vi "Global 1.vi"() -> ()   [LabVIEW 2018]
panel:
  in  "Alarm Message":string
  out "QUIT":bool
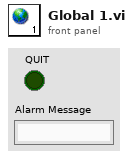
[diagram p1: front panel]
diagram:
